vi "Longest Line Length in Pixels.vi"(10 "String":refnum<vi>) -> (3 "longest line length":i32)   [LabVIEW 2022 SP3]
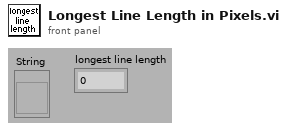
[diagram p1: front panel]
types:
  T1 = enum16{"User-specified Font", "Application Font", "System Font", "Dialog Font"}
  T2 = cluster{"horizontal":enum16{"left", "center", "right"}, "vertical":enum16{"top", "center", "bottom"}}
  T3 = typedef "LVFontTypeDef.ctl" = cluster{"Font Name":string, "Size":u16, "Bold":bool, "Italic":bool, "Underline":bool, "Strikeout":bool, "Color":u32}
  T4 = cluster{"Font Name:":string, "Size":i16, "Strikeout?":bool, "Italic?":bool, "Underline?":bool, "Outline?":bool, "Shadow?":bool, "Bold?":bool}
  T5 = cluster{"left":i16, "top":i16, "right":i16, "bottom":i16}
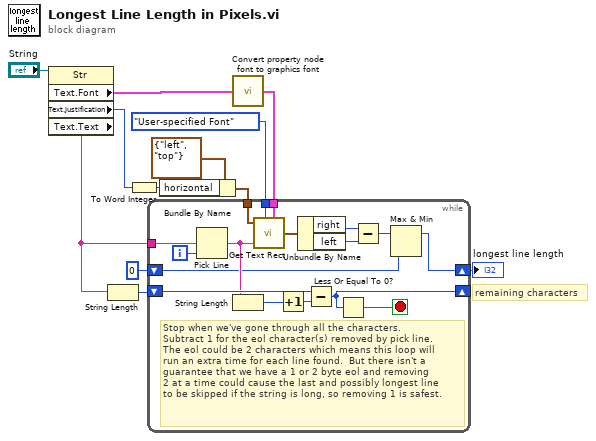
[diagram p0: block diagram]
diagram:
  # "remaining characters"
  n1 = property class="Str"(reference="String") -> ("Text.Font"=w11:T3, "Text.Justification"=w7:enum16{"Left", "Center", "Right"}, "Text.Text"=w3:string)  [unwired: 1 in, 2 out]
  n2 = String Length(string=w3) -> (length=w2:i32)
  n3 = To Word Integer(number=w7) -> (16bit integer=w6:i16)
  n4 = Bundle By Name(cluster=T2 {"horizontal"=enum."left", "vertical"=enum."top"} ("alignment(left, top)"), "horizontal"=w6) -> (w9:T2)
  n5 = call "Convert property node font to graphics font.vi"("String:Text:Font:All Elements font cluster"=w11) -> ("Get Text Rect font cluster"=w10:T4)
  n6 = while {
    tunnel: w9 -> [w29]
    tunnel: w10 -> [w25]
    tunnel: T1."User-specified Font" ("desired font(Application)") -> [w24]
    shift-right: [w15] -> w4
    shift-left: i16 0 -> [w16]
    tunnel: w3 -> [w22]
    shift-right: [w18] -> _
    shift-left: w2 -> [w21]
    i -> [w23]
    stop <- w13 stop-if-true
    # "Stop when we've gone through all the characters.\nSubtract 1 for the eol character(s) removed by pick line.\nThe eol could be 2 characters which means this loop will \nrun an extra time for each line found.  But there isn't a \nguarantee that we have a 1 or 2 byte eol and removing \n2 at a time could cause the last and possibly longest line \nto be skipped if the string is long, so removing 1 is safest."
    n7 = Pick Line(multi-line string=w22, line index=w23) -> (output string=w20:string)  [unwired: 1 in]
    n8 = String Length(string=w20) -> (length=w14:i32)
    n9 = call "Get Text Rect.vi"("alignment(left, top)"=w29, "desired font(Application)"=w24, "text"=w20, "[user-specified font]"=w25) -> ("rect"=w28:T5)  [unwired: 5 in]
    n10 = Increment(x=w14) -> (x+1=w19:i32)
    n11 = Unbundle By Name(w28) -> ("right"=w26:i16, "left"=w27:i16)
    n12 = Subtract(x=w21, y=w19) -> (x-y=w18:i32)
    n13 = Less Or Equal To 0?(x=w18) -> (x <= 0?=w13:bool)
    n14 = Subtract(x=w26, y=w27) -> (x-y=w17:i16)
    n15 = Max & Min(x=w17, y=w16) -> (max(x,y)=w15:i16)  [unwired: 1 out]
  }
  "longest line length" <- w4
